vi "Global_Var_Other.vi"() -> ()   [LabVIEW 2016]
panel:
  in  "Encoder_Dist_Travelled":dbl
  out "Gear_Orientation_Bb_True?":bool
  out "YoYo_In_Range?":bool
  in  "YoYo_Value":dbl
  out "Turret_Pos_Reached?":bool
  out "Shooter_RPM_Reached?":bool
  out "Gear_Rail_Pos_Reached?":bool
  out "Gear_Gate_Pos_Reached?":bool
  out "Gear_Chute_Finished?":bool
  out "Gear_Pusher_Finished?":bool
  in  "Shooter_Limit":dbl
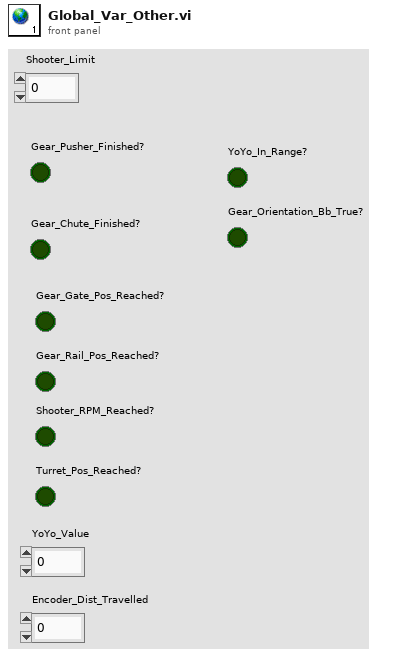
[diagram p1: front panel]
diagram:
